vi "acqComponentsInit_v2.vi"(1 "sCMOS init":cluster{"init":i16, "sCMOS handle":u32}, 2 "XY stage":T3, 3 "Z stage":T2, 4 "Filter wheel init":cluster{"FW Handle":u32, "init?":i16}, 6 "405 nm (aq)":bool=TRUE, 7 "405 filter":u8(ring)=1 items=["460/36 [DAPI]"=1, "525/50 [FITC]"=2, "605/70 [Cy3]"=3, "665/LP [Cy5]"=4, "Empty-1"=5, "Empty-2"=6], 8 "488 nm (aq)":bool=TRUE, 9 "488 filter":u8(ring)=2 items=["460/36 [DAPI]"=1, "525/50 [FITC]"=2, "605/70 [Cy3]"=3, "665/LP [Cy5]"=4, "Empty-1"=5, "Empty-2"=6], 10 "561 nm (aq)":bool=TRUE, 11 "561 filter":u8(ring)=3 items=["460/36 [DAPI]"=1, "525/50 [FITC]"=2, "605/70 [Cy3]"=3, "665/LP [Cy5]"=4, "Empty-1"=5, "Empty-2"=6], 12 "642 nm (aq)":bool=TRUE, 13 "642 filter":u8(ring)=4 items=["460/36 [DAPI]"=1, "525/50 [FITC]"=2, "605/70 [Cy3]"=3, "665/LP [Cy5]"=4, "Empty-1"=5, "Empty-2"=6]) -> (15 "initializedLasers":T1(array[cluster]), 16 "corrCompInit":i16, 17 "initFilters":u8[](array[ring]) items=["460/36 [DAPI]"=1, "525/50 [FITC]"=2, "605/70 [Cy3]"=3, "665/LP [Cy5]"=4, "Empty-1"=5, "Empty-2"=6])   [LabVIEW 2015]
panel:
  in  "LSFM_3 lasers":T1(array[cluster])=[{"Component ID"="405nm", "COM Port"="COM14", "Type "=enum."omicronLuxX", "init"=1}, {"Component ID"="488nm", "COM Port"="COM4", "Type "=enum."omicronLuxX", "init"=1}, {"Component ID"="561nm", "COM Port"="COM27", "Type "=enum."coherentObis", "init"=1}, {"Component ID"="642nm", "COM Port"="COM12", "Type "=enum."omicronLuxX", "init"=1}]
  out "Correct lasers init?":i16=1
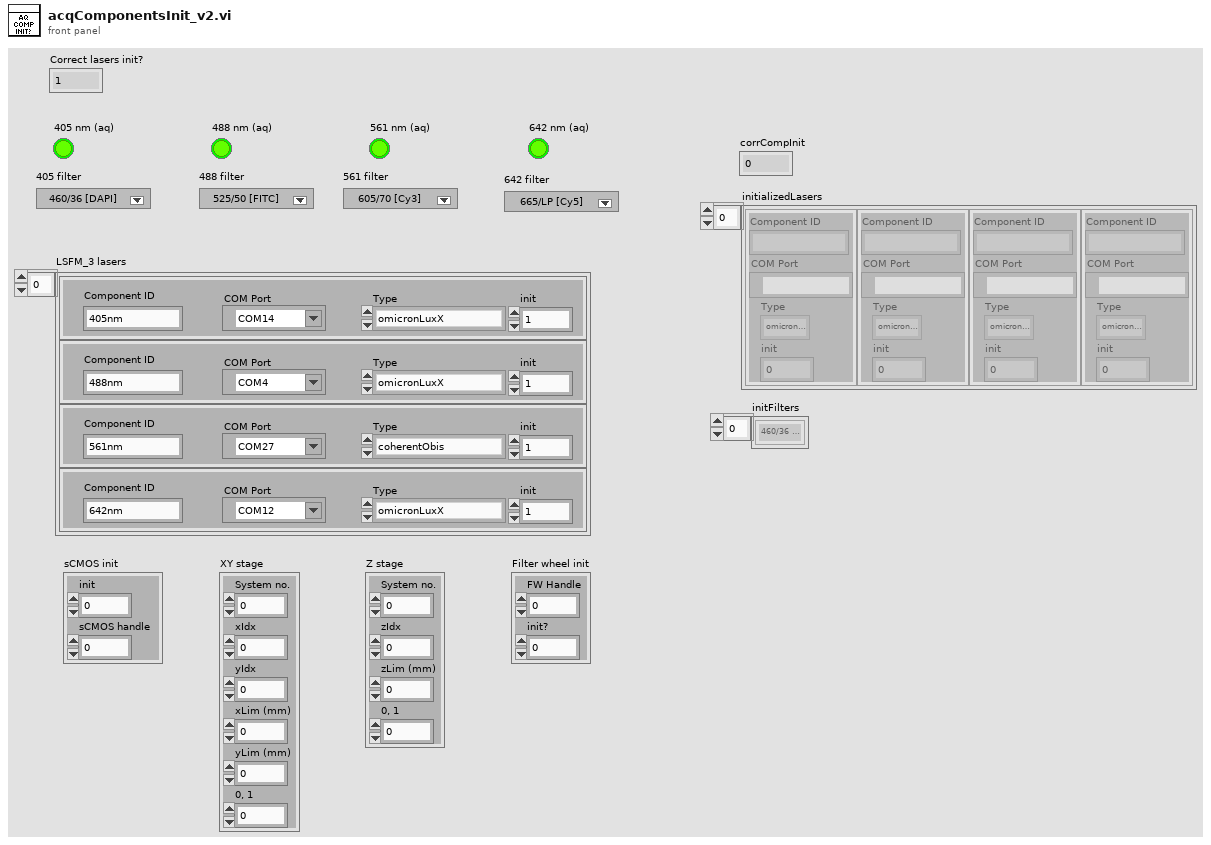
[diagram p1: front panel]
types:
  T1 = cluster{"Component ID":string, "COM Port":refnum<visa-resource-name>, "Type ":enum16{"omicronLuxX", "coherentObis"}, "init":i16}[]
  T2 = cluster{"System no.":i32, "zIdx":i32, "zLim (mm)":dbl, "0, 1":i16}
  T3 = cluster{"System no.":i32, "xIdx":i32, "yIdx":i32, "xLim (mm)":dbl, "yLim (mm)":dbl, "0, 1":i16}
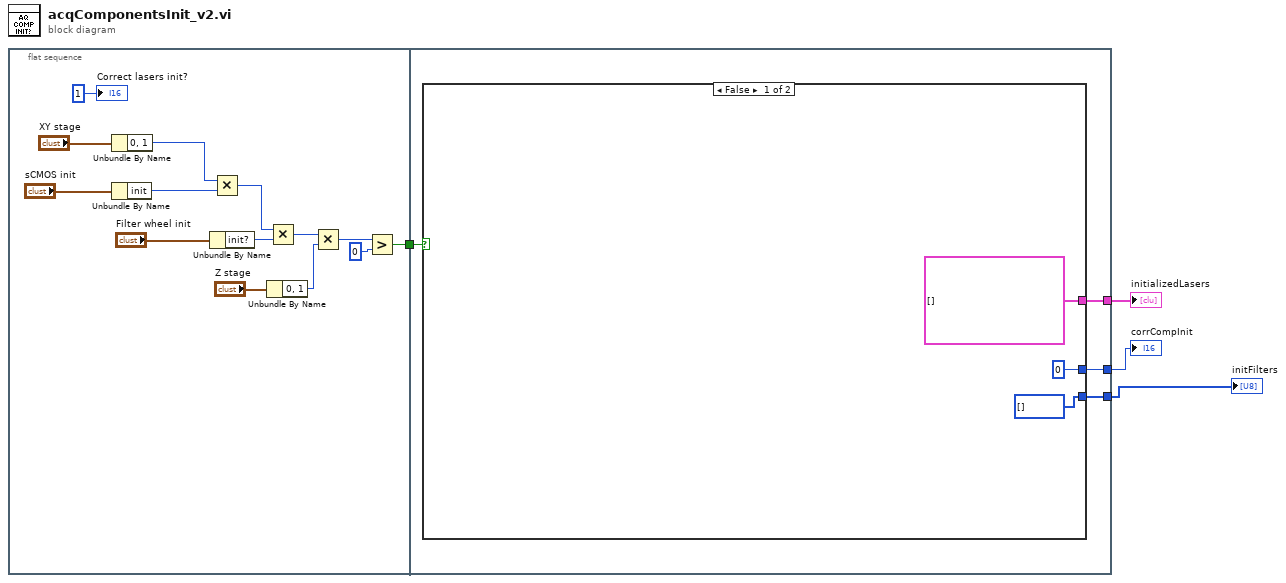
[diagram p0: block diagram]
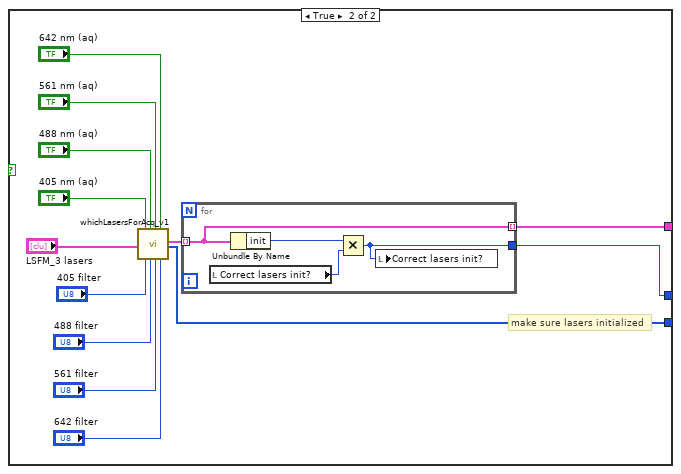
[diagram p2: hidden frame]
diagram:
  n1 = flat-sequence {
    tunnel: [w7] -> w3
    tunnel: [w22] -> w4
    tunnel: w3 -> [w21]
    tunnel: [w20] -> w1
    tunnel: [w19] -> w2
    frame #0 {
      n2 = Unbundle By Name("XY stage") -> ("0, 1"=w14:i16)
      n3 = Unbundle By Name("sCMOS init") -> ("init"=w13:i16)
      n4 = Unbundle By Name("Filter wheel init") -> ("init?"=w11:i16)
      n5 = Multiply(x=w14, y=w13) -> (x*y=w12:i16)
      n6 = Unbundle By Name("Z stage") -> ("0, 1"=w9:i16)
      n7 = Multiply(x=w12, y=w11) -> (x*y=w10:i16)
      n8 = Multiply(x=w10, y=w9) -> (x*y=w8:i16)
      n9 = Greater?(x=w8, y=i16 0) -> (0:w7:bool)
      "Correct lasers init?" <- i16 1 ("Correct lasers init?")
    }
    frame #1 {
      n10 = case shown="False" w21 {
        tunnel: [T1 [] w38] -> w22
        tunnel: [u8[] [] ("Filters") w27] -> w20
        tunnel: [i16 0 w26] -> w19
        frame False {
        }
        frame True {
          # "make sure lasers initialized"
          n11 = call "whichLasersForAcq_v1.vi"("LSFM_3 lasers"="LSFM_3 lasers", "405 nm (aq)"="405 nm (aq)", "405 filter"="405 filter", "488 nm (aq)"="488 nm (aq)", "488 filter"="488 filter", "561 nm (aq)"="561 nm (aq)", "561 filter"="561 filter", "642 nm (aq)"="642 nm (aq)", "642 filter"="642 filter") -> ("Initialized lasers"=w28:T1, "initFilters"=w27:u8[])  [unwired: 9 in]
          n12 = for {
            tunnel: w28 -> [w40] mode=indexing
            tunnel: [w41] -> w26
            tunnel: [w40] -> w38 mode=indexing
            n13 = local read "Correct lasers init?"() -> (w42:i16)
            n14 = Unbundle By Name(w40) -> ("init"=w39:i16)
            n15 = Multiply(x=w39, y=w42) -> (x*y=w41:i16)
            n16 = local write "Correct lasers init?"(w41) -> ()
          }
        }
      }
    }
  }
  "initializedLasers" <- w4
  "corrCompInit" <- w2
  "initFilters" <- w1
